vi "load_presets.vi"(8 "error in (no error)":errorcluster, 11 "ColorOverlay in":refnum<class "ColorOverlay.lvclass">) -> (0 "error out":errorcluster, 3 "ColorOverlay out":refnum<class "ColorOverlay.lvclass">)   [LabVIEW 2010, in "ColorOverlay.lvclass"]
uses:
  ColorOverlay.lvclass
  presets_save_cluster.ctl
  cursor_cluster.ctl
  settings_cluster.ctl
  ColorOverlay.lvclass/ColorOverlay.ctl
panel:
  out "data":T1={"# hot pixels"=0, "# cold pixels"=0, "color lower limit"=16860, "color upper limit"=16711680, "color?"=FALSE, "start color"=[0, 0, 0, 0], "end color"=[0, 0, 0, 0], "array of cursors"=[{"cursor position"=[0.0, 0.0]}, {"cursor position"=[0.0, 0.0]}, {"cursor position"=[0.0, 0.0]}, {"cursor position"=[0.0, 0.0]}]}
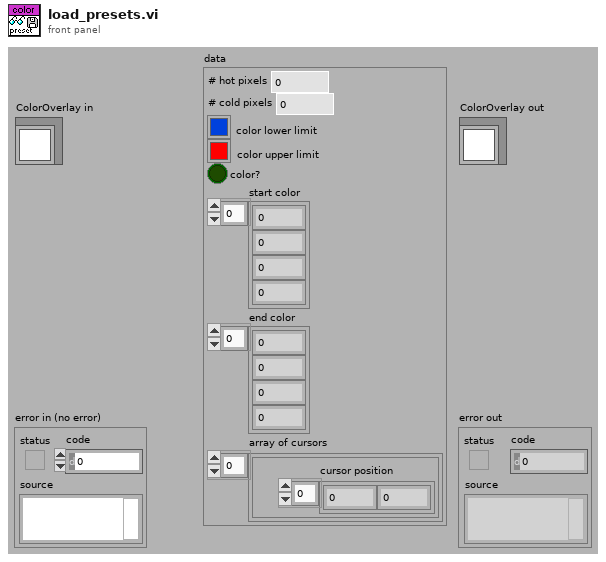
[diagram p1: front panel]
types:
  T1 = typedef "ColorOverlay.lvclass/presets_save_cluster.ctl" = cluster{"# hot pixels":i32, "# cold pixels":i32, "color lower limit":u32, "color upper limit":u32, "color?":bool, "start color":u8[], "end color":u8[], "array of cursors":T2[]}
  T2 = typedef "ColorOverlay.lvclass/cursor_cluster.ctl" = cluster{"cursor position":dbl[]}
  T3 = typedef "ColorOverlay.lvclass/settings_cluster.ctl" = cluster{"# cold pixels":i32, "# hot pixels":i32, "graph editor":cluster{"ramp array out":u32[]}[], "color lower limit":u32, "color upper limit":u32, "color?":bool, "start color":cluster{u8, u8, u8, u8}, "end color":cluster{u8, u8, u8, u8}, "array of cursors":T2[]}
  T4 = enum16{"open", "replace", "create", "open or create", "replace or create", "replace or create with confirmation"}
  T5 = cluster{"start color[0]":u8, "start color[1]":u8, "start color[2]":u8, "start color[3]":u8}
  T6 = cluster{"end color[0]":u8, "end color[1]":u8, "end color[2]":u8, "end color[3]":u8}
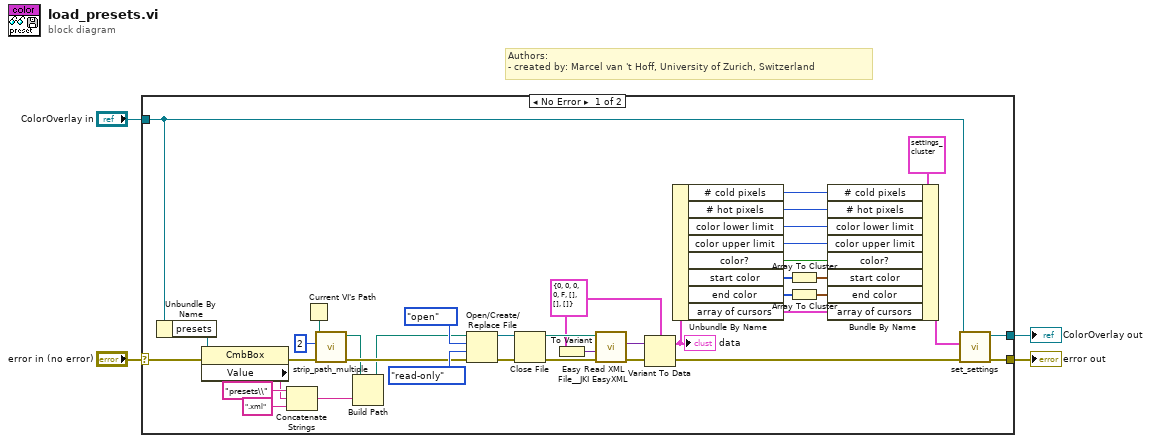
[diagram p0: block diagram]
diagram:
  # "Authors: \n- created by: Marcel van 't Hoff, University of Zurich, Switzerland"
  n1 = case shown="No Error" "error in (no error)" {
    selector: "error in (no error)" -> [w19 w45]
    tunnel: [w33 w45] -> w3
    tunnel: [w35 w44] -> w1
    tunnel: "ColorOverlay in" -> [w21 w44]
    frame No Error {
      w7 = T1 {"# hot pixels"=0, "# cold pixels"=0, "color lower limit"=0, "color upper limit"=0, "color?"=FALSE, "start color"=[], "end color"=[], "array of cursors"=[]} ("presets save cluster")
      n2 = Unbundle By Name(w21) -> ("presets"=w20:refnum<vi>)
      n3 = property class="CmbBox"(reference=w20, error in=w19) -> (error out=w16:errorcluster, "Value"=w11:string)  [unwired: 1 out]
      n4 = Concatenate Strings("presets\\" ("name or relative path"), w11, ".xml" ("string")) -> (w10:string)
      n5 = Current VI's Path() -> (path=w17:path)
      n6 = call "strip_path_multiple.vi"("error in (no error)"=w16, "number of strips"=2, "path in"=w17) -> ("error out"=w15:errorcluster, "path out"=w14:path)  [unwired: 7 in]
      n7 = Build Path(base path=w14, name or relative path=w10) -> (appended path=w9:path)
      n8 = Open/Create/Replace File(file path (use dialog)=w9, error in=w15, operation (0:open)=T4."open", access (0:read/write)=enum16{"read/write", "read-only", "write-only"}."read-only") -> (refnum out=w39:refnum<file>, error out=w42:errorcluster)  [unwired: 2 in, 1 out]
      n9 = Close File(refnum=w39, error in=w42) -> (path=w38:path, error out=w43:errorcluster)
      n10 = To Variant(anything=w7) -> (Variant=w8:variant)
      n11 = call <vilib>:"Easy Read XML File__JKI EasyXML.vi"("error in (no error)"=w43, "LabVIEW Data (Type)"=w8, "XML File Path"=w38) -> ("error out"=w37:errorcluster, "LabVIEW Data"=w36:variant)  [unwired: 6 in, 1 out]
      n12 = Variant To Data(error in=w37, Variant=w36, type=w7) -> (error out=w34:errorcluster, data=w32:T1)
      "data" <- w32
      n13 = Unbundle By Name(w32) -> ("# cold pixels"=w30:i32, "# hot pixels"=w29:i32, "color lower limit"=w28:u32, "color upper limit"=w27:u32, "color?"=w26:bool, "start color"=w25:u8[], "end color"=w24:u8[], "array of cursors"=w23:T2[])
      n14 = Array To Cluster(array=w25) -> (cluster=w6:T5)
      n15 = Array To Cluster(array=w24) -> (cluster=w5:T6)
      n16 = Bundle By Name(cluster=T3 {"# cold pixels"=0, "# hot pixels"=0, "graph editor"=[{"ramp array out"=[0, 1, 2, 3, 4, 5, 6, 7, 8, 9, 10, 11, 12, 13, 14, 15, 16, 17, 18, 19, 20, 21, 22, 23, 24, 25, 26, 27, 28, 29, 30, 31, 32, 33, 34, 35, 36, 37, 38, 39, 40, 41, 42, 43, 44, 45, 46, 47, 48, 49, 50, 51, 52, 53, 54, 55, 56, 57, 58, 59, 60, 61, 62, 63, 64, 65, 66, 67, 68, 69, 70, 71, 72, 73, 74, 75, 76, 77, 78, 79, 80, 81, 82, 83, 84, 85, 86, 87, 88, 89, 90, 91, 92, 93, 94, 95, 96, 97, 98, 99, 100, 101, 102, 103, 104, 105, 106, 107, 108, 109, 110, 111, 112, 113, 114, 115, 116, 117, 118, 119, 120, 121, 122, 123, 124, 125, 126, 127, 126, 125, 124, 123, 122, 121, 120, 119, 118, 117, 116, 115, 114, 113, 112, 111, 110, 109, 108, 107, 106, 105, 104, 103, 102, 101, 100, 99, 98, 97, 96, 95, 95, 94, 93, 92, 91, 90, 89, 88, 87, 86, 85, 84, 83, 82, 81, 80, 79, 78, 77, 76, 75, 74, 73, 72, 71, 70, 69, 68, 67, 66, 65, 64, 63, 62, 61, 60, 59, 58, 57, 56, 55, 54, 53, 52, 51, 50, 49, 48, 47, 46, 45, 44, 43, 42, 41, 40, 39, 38, 37, 36, 35, 34, 33, 32, 32, 31, 30, 29, 28, 27, 26, 25, 24, 23, 22, 21, 20, 19, 18, 17, 16, 15, 14, 13, 12, 11, 10, 9, 8, 7, 6, 5, 4, 3, 2, 1]}, {"ramp array out"=[0, 1, 2, 3, 4, 5, 6, 7, 8, 9, 10, 11, 12, 13, 14, 15, 16, 17, 18, 19, 20, 21, 22, 23, 24, 25, 26, 27, 28, 29, 30, 31, 32, 33, 34, 35, 36, 37, 38, 39, 40, 41, 42, 43, 44, 45, 46, 47, 48, 49, 50, 51, 52, 53, 54, 55, 56, 57, 58, 59, 60, 61, 62, 63, 64, 65, 66, 67, 68, 69, 70, 71, 72, 73, 74, 75, 76, 77, 78, 79, 80, 81, 82, 83, 84, 85, 86, 87, 88, 89, 90, 91, 92, 93, 94, 95, 96, 97, 98, 99, 100, 101, 102, 103, 104, 105, 106, 107, 108, 109, 110, 111, 112, 113, 114, 115, 116, 117, 118, 119, 120, 121, 122, 123, 124, 125, 126, 127, 126, 125, 124, 123, 122, 121, 120, 119, 118, 117, 116, 115, 114, 113, 112, 111, 110, 109, 108, 107, 106, 105, 104, 103, 102, 101, 100, 99, 98, 97, 96, 95, 95, 94, 93, 92, 91, 90, 89, 88, 87, 86, 85, 84, 83, 82, 81, 80, 79, 78, 77, 76, 75, 74, 73, 72, 71, 70, 69, 68, 67, 66, 65, 64, 63, 62, 61, 60, 59, 58, 57, 56, 55, 54, 53, 52, 51, 50, 49, 48, 47, 46, 45, 44, 43, 42, 41, 40, 39, 38, 37, 36, 35, 34, 33, 32, 32, 31, 30, 29, 28, 27, 26, 25, 24, 23, 22, 21, 20, 19, 18, 17, 16, 15, 14, 13, 12, 11, 10, 9, 8, 7, 6, 5, 4, 3, 2, 1]}, {"ramp array out"=[0, 1, 2, 3, 4, 5, 6, 7, 8, 9, 10, 11, 12, 13, 14, 15, 16, 17, 18, 19, 20, 21, 22, 23, 24, 25, 26, 27, 28, 29, 30, 31, 32, 33, 34, 35, 36, 37, 38, 39, 40, 41, 42, 43, 44, 45, 46, 47, 48, 49, 50, 51, 52, 53, 54, 55, 56, 57, 58, 59, 60, 61, 62, 63, 64, 65, 66, 67, 68, 69, 70, 71, 72, 73, 74, 75, 76, 77, 78, 79, 80, 81, 82, 83, 84, 85, 86, 87, 88, 89, 90, 91, 92, 93, 94, 95, 96, 97, 98, 99, 100, 101, 102, 103, 104, 105, 106, 107, 108, 109, 110, 111, 112, 113, 114, 115, 116, 117, 118, 119, 120, 121, 122, 123, 124, 125, 126, 127, 126, 125, 124, 123, 122, 121, 120, 119, 118, 117, 116, 115, 114, 113, 112, 111, 110, 109, 108, 107, 106, 105, 104, 103, 102, 101, 100, 99, 98, 97, 96, 95, 95, 94, 93, 92, 91, 90, 89, 88, 87, 86, 85, 84, 83, 82, 81, 80, 79, 78, 77, 76, 75, 74, 73, 72, 71, 70, 69, 68, 67, 66, 65, 64, 63, 62, 61, 60, 59, 58, 57, 56, 55, 54, 53, 52, 51, 50, 49, 48, 47, 46, 45, 44, 43, 42, 41, 40, 39, 38, 37, 36, 35, 34, 33, 32, 32, 31, 30, 29, 28, 27, 26, 25, 24, 23, 22, 21, 20, 19, 18, 17, 16, 15, 14, 13, 12, 11, 10, 9, 8, 7, 6, 5, 4, 3, 2, 1]}, {"ramp array out"=[0, 1, 2, 3, 4, 5, 6, 7, 8, 9, 10, 11, 12, 13, 14, 15, 16, 17, 18, 19, 20, 21, 22, 23, 24, 25, 26, 27, 28, 29, 30, 31, 32, 33, 34, 35, 36, 37, 38, 39, 40, 41, 42, 43, 44, 45, 46, 47, 48, 49, 50, 51, 52, 53, 54, 55, 56, 57, 58, 59, 60, 61, 62, 63, 64, 65, 66, 67, 68, 69, 70, 71, 72, 73, 74, 75, 76, 77, 78, 79, 80, 81, 82, 83, 84, 85, 86, 87, 88, 89, 90, 91, 92, 93, 94, 95, 96, 97, 98, 99, 100, 101, 102, 103, 104, 105, 106, 107, 108, 109, 110, 111, 112, 113, 114, 115, 116, 117, 118, 119, 120, 121, 122, 123, 124, 125, 126, 127, 126, 125, 124, 123, 122, 121, 120, 119, 118, 117, 116, 115, 114, 113, 112, 111, 110, 109, 108, 107, 106, 105, 104, 103, 102, 101, 100, 99, 98, 97, 96, 95, 95, 94, 93, 92, 91, 90, 89, 88, 87, 86, 85, 84, 83, 82, 81, 80, 79, 78, 77, 76, 75, 74, 73, 72, 71, 70, 69, 68, 67, 66, 65, 64, 63, 62, 61, 60, 59, 58, 57, 56, 55, 54, 53, 52, 51, 50, 49, 48, 47, 46, 45, 44, 43, 42, 41, 40, 39, 38, 37, 36, 35, 34, 33, 32, 32, 31, 30, 29, 28, 27, 26, 25, 24, 23, 22, 21, 20, 19, 18, 17, 16, 15, 14, 13, 12, 11, 10, 9, 8, 7, 6, 5, 4, 3, 2, 1]}], "color lower limit"=16860, "color upper limit"=16711680, "color?"=FALSE, "start color"={0, 0, 255, 0}, "end color"={0, 0, 255, 0}, "array of cursors"=[]} ("settings cluster"), "# cold pixels"=w30, "# hot pixels"=w29, "color lower limit"=w28, "color upper limit"=w27, "color?"=w26, "start color"=w6, "end color"=w5, "array of cursors"=w23) -> (w22:T3)
      n17 = call-dynamic "set_settings.vi"("error in (no error)"=w34, "settings cluster"=w22, "ColorOverlay in"=w21) -> ("error out"=w33:errorcluster, "ColorOverlay out"=w35:refnum<class "ColorOverlay.lvclass">)  [unwired: 7 in]
    }
    frame Error {
    }
  }
  "error out" <- w3
  "ColorOverlay out" <- w1
